vi "Float CDAB.vi"(8 "error in":errorcluster, 10 "starting address":u16=71, 11 "Serial in":refnum<class "MB_Master_Serial.lvclass">) -> (0 "error out":errorcluster, 2 "ABCD":sgl, 3 "Serial out":refnum<class "MB_Master_Serial.lvclass">)   [LabVIEW 2017, in "Akwizycja.lvlib"]
uses:
  Akwizycja.lvlib
  <vilib>/Plasmionique/MB Master/MB_Master_Serial/MB_Master_Serial.lvclass
  D:/Program Files (x86)/National Instruments/LabVIEW 2017/vi.lib/Plasmionique/MB Master/MB_Master/MB_Master.lvclass
  <vilib>/Plasmionique/MB Master/MB Master.lvlib
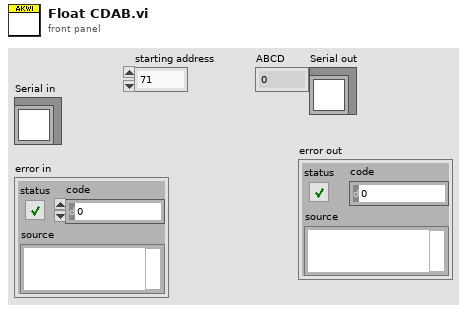
[diagram p1: front panel]
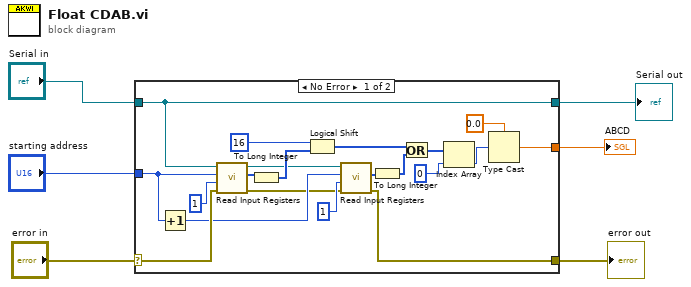
[diagram p0: block diagram]
diagram:
  n1 = case shown="No Error" "error in" {
    selector: "error in" -> [w14 w28]
    tunnel: "Serial in" -> [w17 w27]
    tunnel: "starting address" -> [w16 _]
    tunnel: [w18 _] -> w3
    tunnel: [w11 w28] -> w2
    tunnel: [w17 w27] -> w1
    frame No Error {
      n2 = Increment(x=w16) -> (x+1=w8:u16)
      n3 = call <vilib>:"Read Input Registers.vi"("error in (no error)"=w14, "quantity"=u16 1, "starting address"=w16, "MB session in"=w17) -> ("error out"=w7:errorcluster, "Registers"=w13:u16[], "MB session out"=w9:refnum<class "MB_Master_Serial.lvclass">)  [unwired: 5 in]
      n4 = To Long Integer(number=w13) -> (32bit integer=w24:i32[])
      n5 = Logical Shift(y=16, x=w24) -> (x << y=w21:i32[])
      n6 = call <vilib>:"Read Input Registers.vi"("error in (no error)"=w7, "quantity"=u16 1, "starting address"=w8, "MB session in"=w9) -> ("error out"=w11:errorcluster, "Registers"=w10:u16[])  [unwired: 5 in, 1 out]
      n7 = To Long Integer(number=w10) -> (32bit integer=w20:i32[])
      n8 = Or(x=w21, y=w20) -> (x .or. y?=w22:i32[])
      n9 = Index Array(array=w22, index=0) -> (element=w25:i32)
      n10 = Type Cast(type=sgl 0.0, x=w25) -> (*(type *) &x=w18:sgl)
    }
    frame Error {
    }
  }
  "ABCD" <- w3
  "error out" <- w2
  "Serial out" <- w1
